vi "Create HTTP Request.vi"(5 "httpRequest in":refnum<class "httpRequest.lvclass">, 6 "timeout":i32, 7 "Request Headers":refnum<class "httpHeaders.lvclass">, 8 "error in":errorcluster, 10 "buffer":string, 11 "url":string) -> (0 "error out":errorcluster, 3 "httpRequest out":refnum<class "httpRequest.lvclass">)   [LabVIEW 2020, in "httpClient.lvlib" / "httpRequest.lvclass"]
uses:
  httpRequest.lvclass
  httpHeaders/httpHeaders.lvclass
  httpRequest.lvclass/httpRequest.ctl
  Write url.vi
  Write buffer.vi
  Write timeout.vi
  Read buffer.vi
  Write httpHeaders.vi
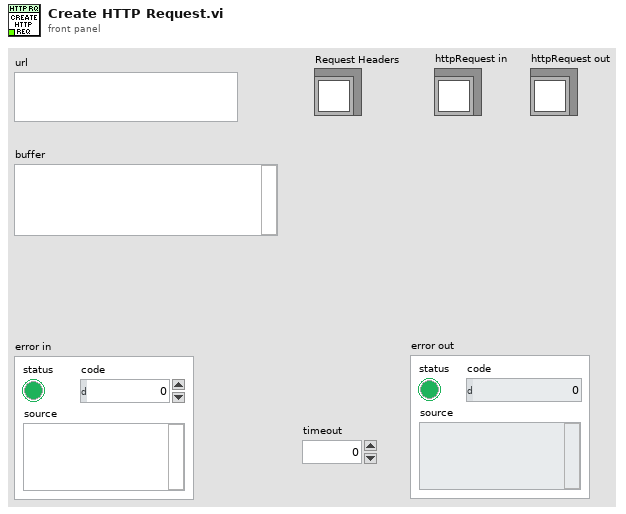
[diagram p1: front panel]
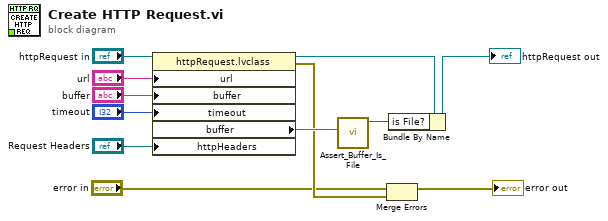
[diagram p0: block diagram]
diagram:
  n1 = property class="httpRequest.lvclass"(reference="httpRequest in", "url"="url", "buffer"="buffer", "timeout"="timeout", "httpHeaders"="Request Headers") -> (reference out=w9:refnum<class "httpRequest.lvclass">, error out=w3:errorcluster, "buffer"=w5:string)  [unwired: 1 in]
  n2 = call "Assert_Buffer_Is_File.vi"("buffer"=w5) -> ("is File?"=w10:bool)  [unwired: 9 in, 1 out]
  n3 = Merge Errors("error in", w3) -> (→"error out":errorcluster)
  n4 = Bundle By Name(cluster=w9, "is File?"=w10) -> (→"httpRequest out":refnum<class "httpRequest.lvclass">)
